vi "Cycling_No_DAQ_Tasks_RT - cOver100.vi"() -> ()   [LabVIEW 2020]
uses:
  Device-Interface-Layer/stop button3.vi
  Device-Interface-Layer/stop button2.vi
  Device-Interface-Layer/stop button1.vi
panel:
  out "Battery 1 Temp":dbl(graph)
  out "Battery 1 Strain":dbl(graph)
  out "Battery 1 Voltage":dbl(graph)
  out "Battery 1 Current":dbl(graph)
  out "Battery 2 Temp":dbl(graph)
  out "Battery 2 Strain":dbl(graph)
  out "Battery 2 Voltage":dbl(graph)
  out "Battery 2 Current":dbl(graph)
  out "Battery 3 Current":dbl(graph)
  out "Battery 3 Voltage":dbl(graph)
  out "Battery 3 Strain":dbl(graph)
  out "Boolean":bool=TRUE
  out "Battery 3 Temp":dbl(graph)
  out "PS Visa Out 3":refnum<visa-resource-name>
  out "PS error out 3":errorcluster
  in  "PS error in 3":errorcluster caption="PS error in (no error)"
  out "PS Visa Out 2":refnum<visa-resource-name>
  out "PS error out 2":errorcluster
  in  "PS error in 2":errorcluster caption="PS error in (no error)"
  out "PS error out":errorcluster
  out "PS Visa Out":refnum<visa-resource-name>
  in  "PS error in":errorcluster caption="PS error in (no error)"
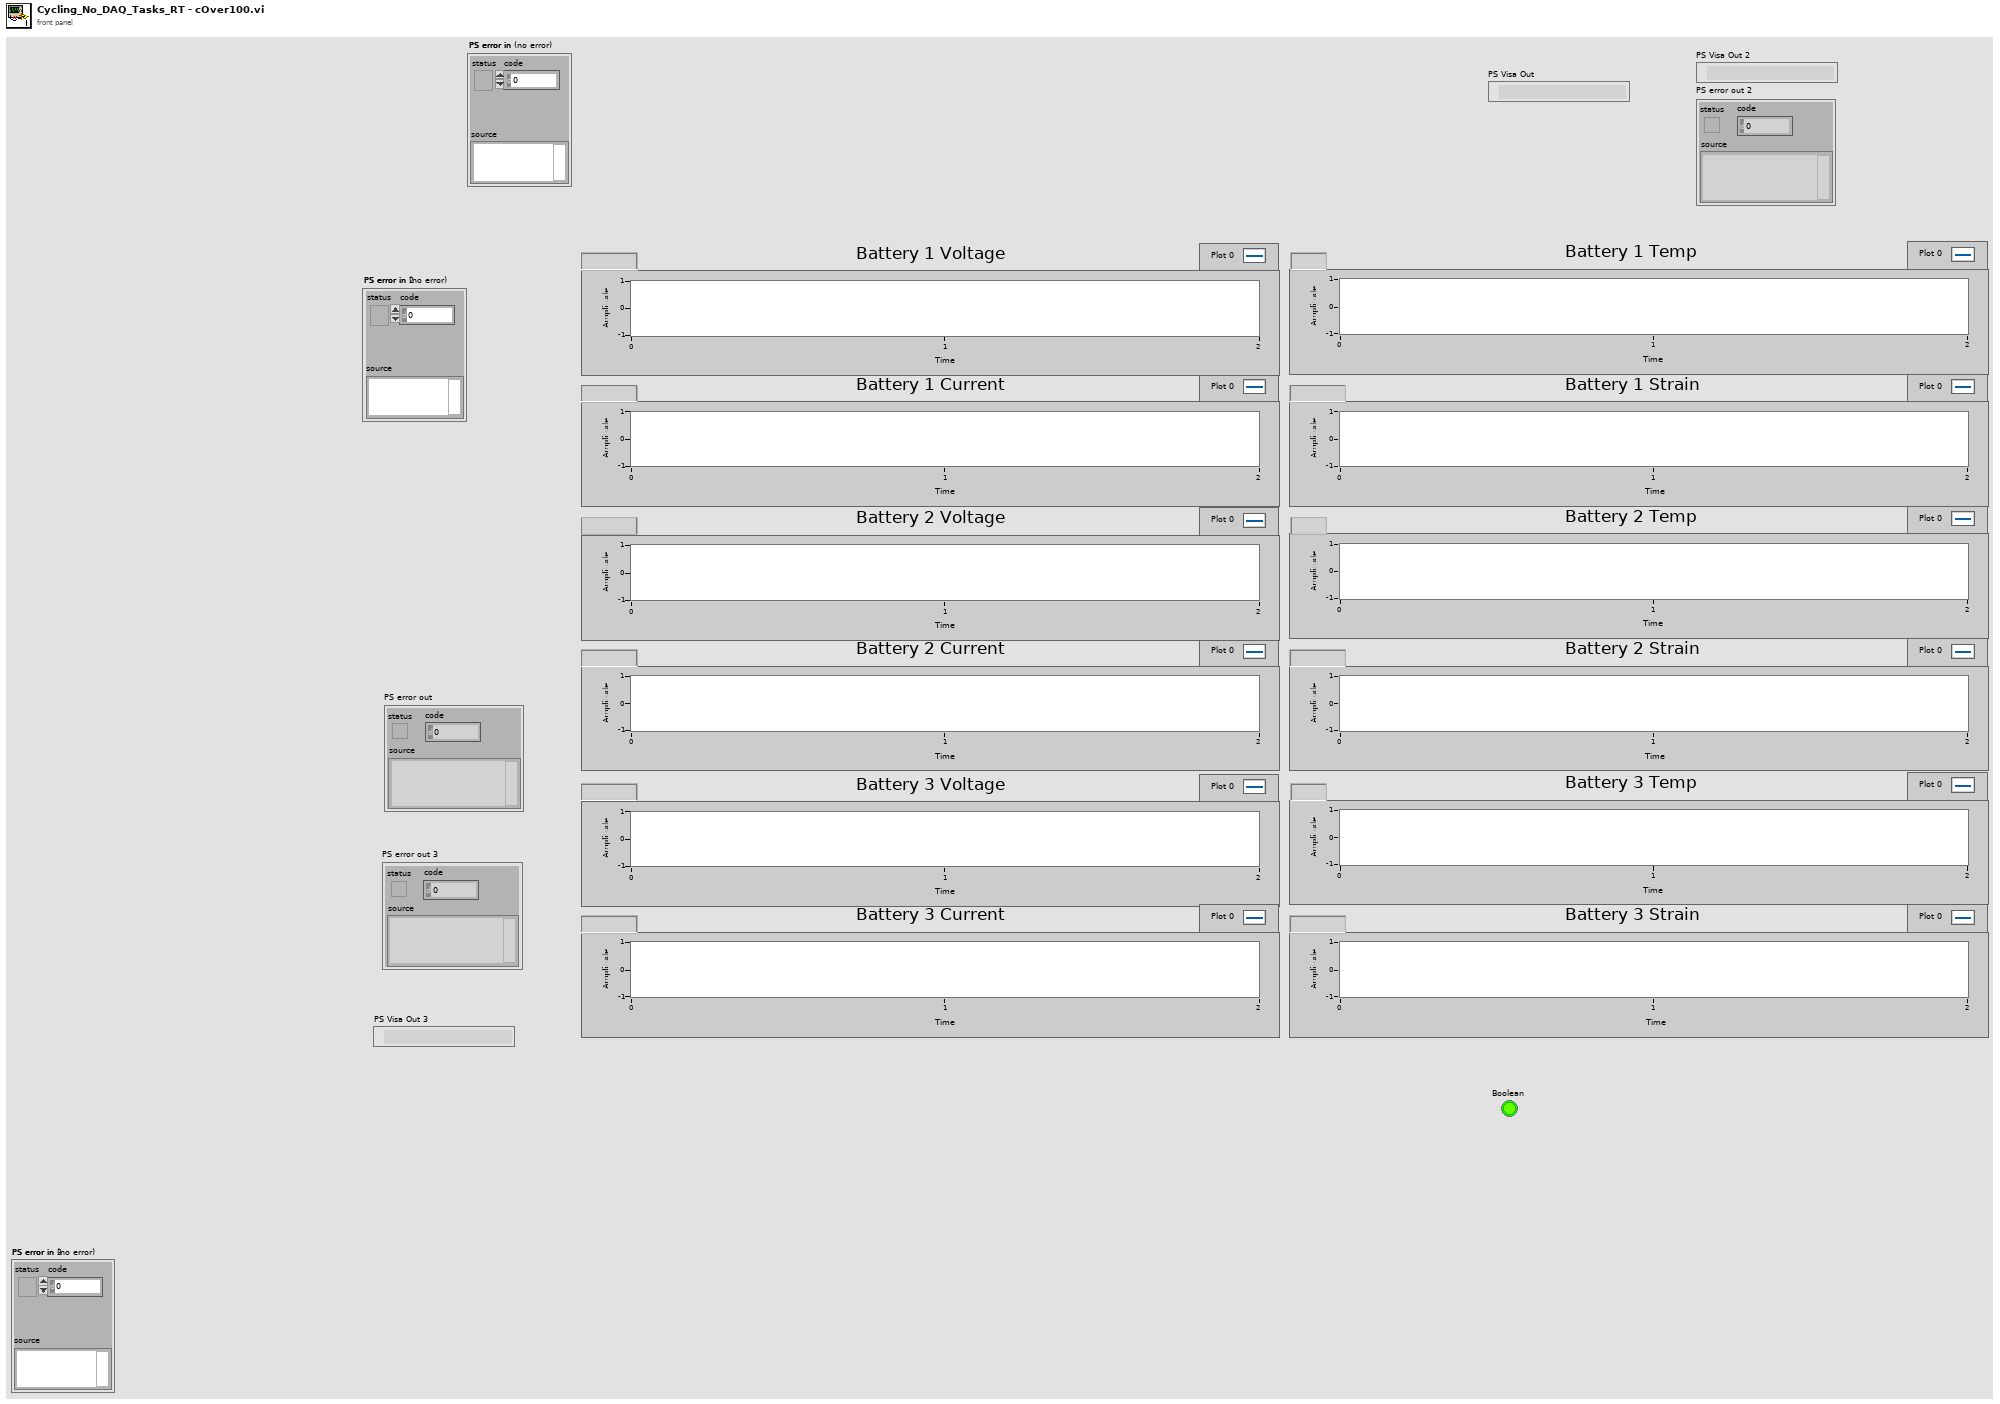
[diagram p1: front panel]
types:
  T1 = enum16{"\"30Q\"", "\"40T\"", "\"2P30Q\"", "\"3P30Q\"", "\"Nissan Leaf\""}
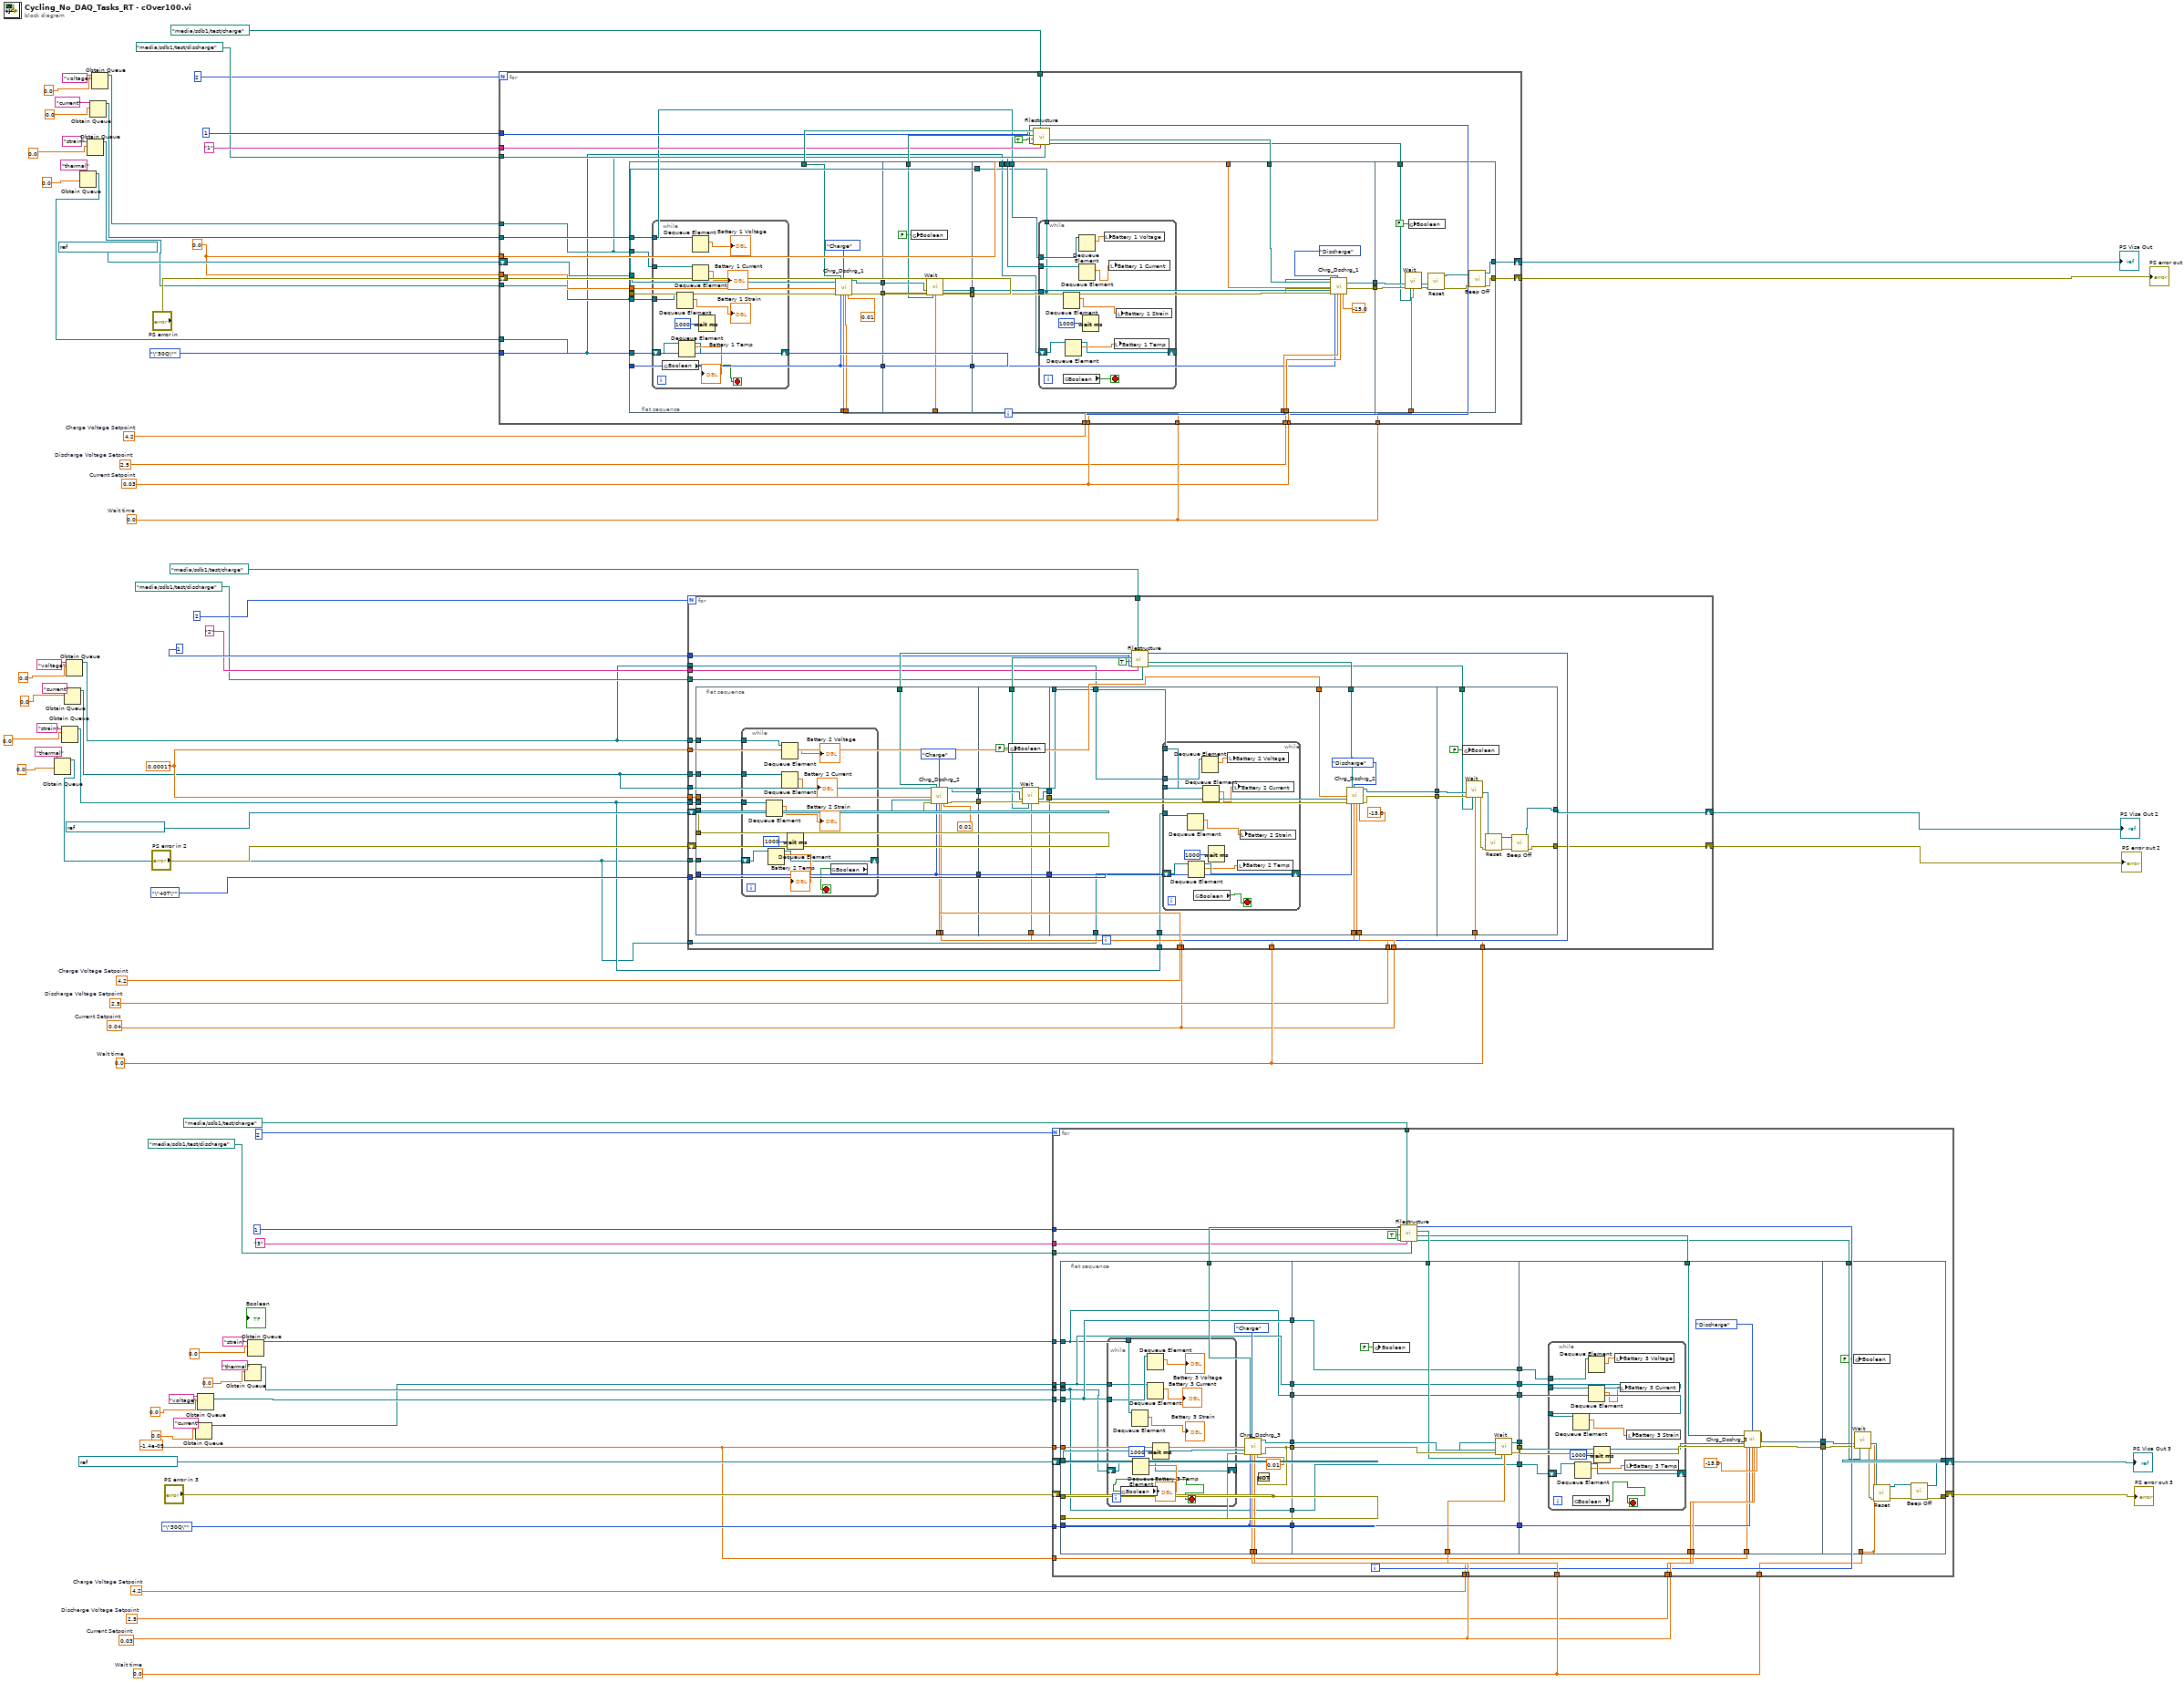
[diagram p0: block diagram]
diagram:
  w3 = -1.4e-05 ("Strain Offset")
  w38 = 0.00017 ("Strain Offset")
  w39 = 2.5  # Discharge Voltage Setpoint
  w42 = 0.0  # Wait time
  w40 = 0.03  # Current Setpoint
  w41 = 4.2  # Charge Voltage Setpoint
  w45 = 2.5  # Discharge Voltage Setpoint
  w46 = 0.0  # Wait time
  w44 = 0.04  # Current Setpoint
  w43 = 4.2  # Charge Voltage Setpoint
  w47 = 2.5  # Discharge Voltage Setpoint
  w50 = 0.0 ("Strain Offset")
  w51 = 0.0  # Wait time
  w49 = 0.03  # Current Setpoint
  w48 = 4.2  # Charge Voltage Setpoint
  n1 = Obtain Queue(name (unnamed)="thermal", element data type=0.0) -> (queue out=w4:refnum<queue>)  [unwired: 3 in, 2 out]
  n2 = Obtain Queue(name (unnamed)="strain", element data type=0.0) -> (queue out=w5:refnum<queue>)  [unwired: 3 in, 2 out]
  n3 = Obtain Queue(name (unnamed)="current", element data type=0.0) -> (queue out=w6:refnum<queue>)  [unwired: 3 in, 2 out]
  n4 = Obtain Queue(name (unnamed)="voltage", element data type=0.0) -> (queue out=w7:refnum<queue>)  [unwired: 3 in, 2 out]
  n5 = Obtain Queue(name (unnamed)="thermal", element data type=0.0) -> (queue out=w8:refnum<queue>)  [unwired: 3 in, 2 out]
  n6 = Obtain Queue(name (unnamed)="strain", element data type=0.0) -> (queue out=w9:refnum<queue>)  [unwired: 3 in, 2 out]
  n7 = Obtain Queue(name (unnamed)="current", element data type=0.0) -> (queue out=w10:refnum<queue>)  [unwired: 3 in, 2 out]
  n8 = Obtain Queue(name (unnamed)="voltage", element data type=0.0) -> (queue out=w11:refnum<queue>)  [unwired: 3 in, 2 out]
  n9 = Obtain Queue(name (unnamed)="current", element data type=0.0) -> (queue out=w30:refnum<queue>)  [unwired: 3 in, 2 out]
  n10 = Obtain Queue(name (unnamed)="voltage", element data type=0.0) -> (queue out=w31:refnum<queue>)  [unwired: 3 in, 2 out]
  n11 = Obtain Queue(name (unnamed)="thermal", element data type=0.0) -> (queue out=w36:refnum<queue>)  [unwired: 3 in, 2 out]
  n12 = Obtain Queue(name (unnamed)="strain", element data type=0.0) -> (queue out=w34:refnum<queue>)  [unwired: 3 in, 2 out]
  n13 = for {
    N: 2 ("Number of Cycles") -> [_]
    tunnel: T1."\"30Q\"" ("Battery Type") -> [w106]
    tunnel: w48 -> [w105]
    tunnel: w49 -> [w104]
    tunnel: w51 -> [w92]
    shift-right: [w83] -> w78
    shift-left: refnum<visa-resource-name> "TCPIP0::192.168.0.246::inst0::INSTR" ("PS VISA in") -> [w108]
    shift-right: [w82] -> w79
    shift-left: "PS error in" -> [w107]
    tunnel: 1 ("Starting Cycle") -> [w98]
    tunnel: "1" ("Batteryname") -> [w96]
    tunnel: path "/media/sdb1/test/discharge" ("Discharge filepath") -> [w95]
    tunnel: path "/media/sdb1/test/charge" ("Charge filepath") -> [w94]
    tunnel: w51 -> [w93]
    tunnel: w50 -> [w91]
    tunnel: w50 -> [w90]
    tunnel: w49 -> [w89]
    tunnel: w47 -> [w88]
    tunnel: w11 -> [w87]
    tunnel: w10 -> [w86]
    tunnel: w9 -> [w85]
    tunnel: w8 -> [w84]
    i -> [w99]
    n14 = flat-sequence {
      tunnel: w108 -> [w125]
      tunnel: w107 -> [w126]
      tunnel: w106 -> [w127]
      tunnel: w105 -> [w122]
      tunnel: [w129] -> w116
      tunnel: [w121] -> w115
      tunnel: [w127] -> w114
      tunnel: w103 -> [w130]
      tunnel: w91 -> [w124]
      tunnel: w89 -> [w123]
      tunnel: w87 -> [w120]
      tunnel: w86 -> [w119]
      tunnel: w85 -> [w118]
      tunnel: w84 -> [w117]
      tunnel: w116 -> [w149]
      tunnel: w115 -> [w148]
      tunnel: [w145] -> w113
      tunnel: [w146] -> w112
      tunnel: w114 -> [w150]
      tunnel: [w150] -> w111
      tunnel: w102 -> [w147]
      tunnel: w92 -> [w144]
      tunnel: w113 -> [w160]
      tunnel: w112 -> [w161]
      tunnel: w111 -> [w162]
      tunnel: w88 -> [w163]
      tunnel: w104 -> [w164]
      tunnel: w101 -> [w159]
      tunnel: [w157] -> w110
      tunnel: [w156] -> w109
      tunnel: w90 -> [w155]
      tunnel: w87 -> [w154]
      tunnel: w86 -> [w153]
      tunnel: w85 -> [w152]
      tunnel: w84 -> [w151]
      tunnel: w100 -> [w182]
      tunnel: w110 -> [w187]
      tunnel: w109 -> [w186]
      tunnel: w93 -> [w183]
      tunnel: [w178] -> w83
      tunnel: [w177] -> w82
      frame #0 {
        n15 = while {
          shift-right: [w140] -> _
          shift-left: w117 -> [w139]
          tunnel: w119 -> [w137]
          tunnel: w120 -> [w134]
          tunnel: w118 -> [w133]
          stop <- w132 stop-if-true
          n16 = global read "stop button1.vi" "Boolean"() -> (w132:bool)
          n17 = Dequeue Element(queue=w133) -> (element=→"Battery 1 Strain":dbl)  [unwired: 2 in, 3 out]
          n18 = Dequeue Element(queue=w139) -> (queue out=w140:refnum<queue>, element=→"Battery 1 Temp":dbl)  [unwired: 2 in, 2 out]
          n19 = Dequeue Element(queue=w134) -> (element=→"Battery 1 Voltage":dbl)  [unwired: 2 in, 3 out]
          n20 = Dequeue Element(queue=w137) -> (element=→"Battery 1 Current":dbl)  [unwired: 2 in, 3 out]
          n21 = Wait (ms)(milliseconds to wait=1000) -> ()  [unwired: 1 out]
        }
        n22 = call "Chrg_Dschrg_1.vi"("Strain Offset"=w124, "PS VISA in"=w125, "PS error in"=w126, "CyclePath"=w130, "Battery Type"=w127, "Charge/discharge"=enum8{"Charge", "Discharge"}."Charge", "Charge/Discharge Voltage Setpoint"=w122, "Current Setpoint"=w123, "Current Cutoff"=0.01) -> ("PS VISA out"=w129:refnum<visa-resource-name>, "PS error out"=w121:errorcluster)  [unwired: 9 in]
      }
      frame #1 {
        n23 = global write "stop button1.vi" "Boolean"(FALSE ("Boolean")) -> ()
        n24 = call "Wait.vi"("PS VISA in"=w149, "PS error in"=w148, "Wait Filepath"=w147, "Wait time"=w144) -> ("PS Visa Out"=w145:refnum<visa-resource-name>, "PS error out"=w146:errorcluster)  [unwired: 10 in]
      }
      frame #2 {
        n25 = while {
          shift-right: [w175] -> _
          shift-left: w151 -> [w174]
          tunnel: [w167] -> _
          tunnel: w153 -> [w173]
          tunnel: w154 -> [w168]
          tunnel: w152 -> [w167]
          stop <- w166 stop-if-true
          n26 = Dequeue Element(queue=w167) -> (element=w170:dbl)  [unwired: 2 in, 3 out]
          n27 = global read "stop button1.vi" "Boolean"() -> (w166:bool)
          n28 = Dequeue Element(queue=w174) -> (queue out=w175:refnum<queue>, element=w169:dbl)  [unwired: 2 in, 2 out]
          n29 = Dequeue Element(queue=w168) -> (element=w172:dbl)  [unwired: 2 in, 3 out]
          n30 = Dequeue Element(queue=w173) -> (element=w171:dbl)  [unwired: 2 in, 3 out]
          n31 = Wait (ms)(milliseconds to wait=1000) -> ()  [unwired: 1 out]
          n32 = local write "Battery 1 Voltage"(w172) -> ()
          n33 = local write "Battery 1 Current"(w171) -> ()
          n34 = local write "Battery 1 Temp"(w169) -> ()
          n35 = local write "Battery 1 Strain"(w170) -> ()
        }
        n36 = call "Chrg_Dschrg_1.vi"("Strain Offset"=w155, "PS VISA in"=w160, "PS error in"=w161, "CyclePath"=w159, "Battery Type"=w162, "Charge/discharge"=enum8{"Charge", "Discharge"}."Discharge", "Charge/Discharge Voltage Setpoint"=w163, "Current Setpoint"=w164, "Current Cutoff"=-15.0) -> ("PS VISA out"=w157:refnum<visa-resource-name>, "PS error out"=w156:errorcluster)  [unwired: 9 in]
      }
      frame #3 {
        n37 = call "Wait.vi"("PS VISA in"=w187, "PS error in"=w186, "Wait Filepath"=w182, "Wait time"=w183) -> ("PS Visa Out"=w185:refnum<visa-resource-name>, "PS error out"=w184:errorcluster)  [unwired: 10 in]
        n38 = global write "stop button1.vi" "Boolean"(FALSE ("Boolean")) -> ()
        n39 = call "Reset.vi"("error in"=w184, "VISA resource name"=w185) -> ("error out"=w179:errorcluster, "VISA resource name out"=w180:refnum<visa-resource-name>)  [unwired: 8 in]
        n40 = call "Beep Off.vi"("error in"=w179, "VISA resource name"=w180) -> ("error out"=w177:errorcluster, "VISA resource name out"=w178:refnum<visa-resource-name>)  [unwired: 8 in]
      }
    }
    n41 = call "Filestructure.vi"("Discharge filepath"=w95, "Batteryname"=w96, "Charge filepath"=w94, "For loop i"=w99, "In for loop"=TRUE, "Starting Cycle"=w98) -> ("DischargeWaitPath"=w100:path, "DischargeCyclePath"=w101:path, "ChargeWaitPath"=w102:path, "ChargeCyclePath"=w103:path)  [unwired: 1 in, 1 out]
  }
  "PS error out" <- w79
  "PS Visa Out" <- w78
  n42 = for {
    N: 2 ("Number of Cycles") -> [_]
    tunnel: T1."\"40T\"" ("Battery Type") -> [w216]
    tunnel: w44 -> [w215]
    tunnel: w44 -> [w214]
    shift-right: [w209] -> w68
    shift-left: refnum<visa-resource-name> "TCPIP0::192.168.0.247::inst0::INSTR" ("PS VISA in") -> [w218]
    shift-right: [w202] -> w69
    shift-left: "PS error in 2" -> [w217]
    tunnel: 1 ("Starting Cycle") -> [w207]
    tunnel: "2" ("Batteryname 2") -> [w205]
    tunnel: path "/media/sdb1/test/discharge" ("Discharge filepath") -> [w204]
    tunnel: path "/media/sdb1/test/charge" ("Charge filepath") -> [w203]
    tunnel: w46 -> [w201]
    tunnel: w46 -> [w200]
    tunnel: w45 -> [w199]
    tunnel: w43 -> [w198]
    tunnel: w38 -> [w197]
    tunnel: w38 -> [w196]
    tunnel: w7 -> [w195]
    tunnel: w6 -> [w194]
    tunnel: w5 -> [w193]
    tunnel: w4 -> [w192]
    tunnel: w7 -> [w191]
    tunnel: w6 -> [w190]
    tunnel: w5 -> [w189]
    tunnel: w4 -> [w188]
    i -> [w208]
    n43 = flat-sequence {
      tunnel: w218 -> [w235]
      tunnel: w217 -> [w236]
      tunnel: w216 -> [w237]
      tunnel: w215 -> [w238]
      tunnel: [w234] -> w226
      tunnel: [w231] -> w225
      tunnel: [w237] -> w224
      tunnel: w213 -> [w240]
      tunnel: w198 -> [w233]
      tunnel: w197 -> [w232]
      tunnel: w195 -> [w230]
      tunnel: w194 -> [w229]
      tunnel: w193 -> [w228]
      tunnel: w192 -> [w227]
      tunnel: w226 -> [w259]
      tunnel: w225 -> [w258]
      tunnel: [w254] -> w223
      tunnel: [w255] -> w222
      tunnel: w224 -> [w260]
      tunnel: [w260] -> w221
      tunnel: w212 -> [w257]
      tunnel: w200 -> [w256]
      tunnel: w223 -> [w270]
      tunnel: w222 -> [w271]
      tunnel: w221 -> [w272]
      tunnel: w199 -> [w273]
      tunnel: w214 -> [w274]
      tunnel: w211 -> [w269]
      tunnel: [w267] -> w220
      tunnel: [w266] -> w219
      tunnel: w196 -> [w265]
      tunnel: w191 -> [w264]
      tunnel: w190 -> [w263]
      tunnel: w189 -> [w262]
      tunnel: w188 -> [w261]
      tunnel: w210 -> [w292]
      tunnel: w220 -> [w297]
      tunnel: w219 -> [w296]
      tunnel: w201 -> [w293]
      tunnel: [w290] -> w209
      tunnel: [w287] -> w202
      frame #0 {
        n44 = while {
          shift-right: [w250] -> _
          shift-left: w227 -> [w249]
          tunnel: w229 -> [w247]
          tunnel: w230 -> [w244]
          tunnel: w228 -> [w243]
          stop <- w242 stop-if-true
          n45 = Dequeue Element(queue=w243) -> (element=→"Battery 2 Strain":dbl)  [unwired: 2 in, 3 out]
          n46 = Dequeue Element(queue=w249) -> (queue out=w250:refnum<queue>, element=→"Battery 2 Temp":dbl)  [unwired: 2 in, 2 out]
          n47 = Dequeue Element(queue=w244) -> (element=→"Battery 2 Voltage":dbl)  [unwired: 2 in, 3 out]
          n48 = Dequeue Element(queue=w247) -> (element=→"Battery 2 Current":dbl)  [unwired: 2 in, 3 out]
          n49 = Wait (ms)(milliseconds to wait=1000) -> ()  [unwired: 1 out]
          n50 = global read "stop button2.vi" "Boolean"() -> (w242:bool)
        }
        n51 = call "Chrg_Dschrg_2.vi"("Strain Offset"=w232, "PS VISA in"=w235, "PS error in"=w236, "CyclePath"=w240, "Battery Type"=w237, "Charge/discharge"=enum8{"Charge", "Discharge"}."Charge", "Charge/Discharge Voltage Setpoint"=w233, "Current Setpoint"=w238, "Current Cutoff"=0.01) -> ("PS VISA out"=w234:refnum<visa-resource-name>, "PS error out"=w231:errorcluster)  [unwired: 9 in]
      }
      frame #1 {
        n52 = global write "stop button2.vi" "Boolean"(FALSE ("Boolean")) -> ()
        n53 = call "Wait.vi"("PS VISA in"=w259, "PS error in"=w258, "Wait Filepath"=w257, "Wait time"=w256) -> ("PS Visa Out"=w254:refnum<visa-resource-name>, "PS error out"=w255:errorcluster)  [unwired: 10 in]
      }
      frame #2 {
        n54 = while {
          shift-right: [w285] -> _
          shift-left: w261 -> [w284]
          tunnel: w262 -> [w283]
          tunnel: [w277] -> _
          tunnel: w264 -> [w278]
          tunnel: w263 -> [w277]
          stop <- w276 stop-if-true
          n55 = Dequeue Element(queue=w283) -> (element=w280:dbl)  [unwired: 2 in, 3 out]
          n56 = Dequeue Element(queue=w284) -> (queue out=w285:refnum<queue>, element=w279:dbl)  [unwired: 2 in, 2 out]
          n57 = global read "stop button2.vi" "Boolean"() -> (w276:bool)
          n58 = Dequeue Element(queue=w278) -> (element=w282:dbl)  [unwired: 2 in, 3 out]
          n59 = Dequeue Element(queue=w277) -> (element=w281:dbl)  [unwired: 2 in, 3 out]
          n60 = Wait (ms)(milliseconds to wait=1000) -> ()  [unwired: 1 out]
          n61 = local write "Battery 2 Voltage"(w282) -> ()
          n62 = local write "Battery 2 Current"(w281) -> ()
          n63 = local write "Battery 2 Temp"(w279) -> ()
          n64 = local write "Battery 2 Strain"(w280) -> ()
        }
        n65 = call "Chrg_Dschrg_2.vi"("Strain Offset"=w265, "PS VISA in"=w270, "PS error in"=w271, "CyclePath"=w269, "Battery Type"=w272, "Charge/discharge"=enum8{"Charge", "Discharge"}."Discharge", "Charge/Discharge Voltage Setpoint"=w273, "Current Setpoint"=w274, "Current Cutoff"=-15.0) -> ("PS VISA out"=w267:refnum<visa-resource-name>, "PS error out"=w266:errorcluster)  [unwired: 9 in]
      }
      frame #3 {
        n66 = global write "stop button2.vi" "Boolean"(FALSE ("Boolean")) -> ()
        n67 = call "Wait.vi"("PS VISA in"=w297, "PS error in"=w296, "Wait Filepath"=w292, "Wait time"=w293) -> ("PS Visa Out"=w295:refnum<visa-resource-name>, "PS error out"=w294:errorcluster)  [unwired: 10 in]
        n68 = call "Reset.vi"("error in"=w294, "VISA resource name"=w295) -> ("error out"=w288:errorcluster, "VISA resource name out"=w289:refnum<visa-resource-name>)  [unwired: 8 in]
        n69 = call "Beep Off.vi"("error in"=w288, "VISA resource name"=w289) -> ("error out"=w287:errorcluster, "VISA resource name out"=w290:refnum<visa-resource-name>)  [unwired: 8 in]
      }
    }
    n70 = call "Filestructure.vi"("Discharge filepath"=w204, "Batteryname"=w205, "Charge filepath"=w203, "For loop i"=w208, "In for loop"=TRUE, "Starting Cycle"=w207) -> ("DischargeWaitPath"=w210:path, "DischargeCyclePath"=w211:path, "ChargeWaitPath"=w212:path, "ChargeCyclePath"=w213:path)  [unwired: 1 in, 1 out]
  }
  "PS error out 2" <- w69
  "PS Visa Out 2" <- w68
  n71 = for {
    N: 2 ("Number of Cycles") -> [_]
    tunnel: T1."\"30Q\"" ("Battery Type") -> [w331]
    tunnel: w40 -> [w330]
    tunnel: w40 -> [w329]
    tunnel: w42 -> [w324]
    shift-right: [w323] -> w58
    shift-left: refnum<visa-resource-name> "TCPIP0::192.168.0.248::inst0::INSTR" ("PS VISA in") -> [w332]
    shift-right: [w316] -> w59
    shift-left: "PS error in 3" -> [w311]
    tunnel: 1 ("Starting Cycle") -> [w321]
    tunnel: "3" ("Batteryname 3") -> [w319]
    tunnel: path "/media/sdb1/test/discharge" ("Discharge filepath") -> [w318]
    tunnel: path "/media/sdb1/test/charge" ("Charge filepath") -> [w317]
    tunnel: w42 -> [w315]
    tunnel: w41 -> [w314]
    tunnel: w39 -> [w313]
    tunnel: w3 -> [w312]
    tunnel: w36 -> [w310]
    tunnel: w34 -> [w309]
    tunnel: w31 -> [w308]
    tunnel: w30 -> [w307]
    tunnel: w3 -> [w298]
    i -> [w322]
    n72 = flat-sequence {
      tunnel: w332 -> [w348]
      tunnel: w311 -> [w349]
      tunnel: w331 -> [w350]
      tunnel: w330 -> [w351]
      tunnel: [w353] -> w340
      tunnel: [w345] -> w339
      tunnel: [w350] -> w338
      tunnel: w328 -> [w354]
      tunnel: w314 -> [w347]
      tunnel: w312 -> [w346]
      tunnel: w311 -> [_]
      tunnel: w310 -> [w341]
      tunnel: w309 -> [w342]
      tunnel: w308 -> [w344]
      tunnel: w307 -> [w343]
      tunnel: [w344] -> w306
      tunnel: [w343] -> w305
      tunnel: [w342] -> w304
      tunnel: [w341] -> w303
      tunnel: w340 -> [w377]
      tunnel: w339 -> [w376]
      tunnel: [w372] -> w337
      tunnel: [w373] -> w336
      tunnel: w338 -> [w378]
      tunnel: [w378] -> w335
      tunnel: w327 -> [w375]
      tunnel: w324 -> [w374]
      tunnel: w306 -> [w371]
      tunnel: w305 -> [w370]
      tunnel: w304 -> [w369]
      tunnel: w303 -> [w368]
      tunnel: [w371] -> w302
      tunnel: [w370] -> w301
      tunnel: [w369] -> w300
      tunnel: [w368] -> w299
      tunnel: w337 -> [w388]
      tunnel: w336 -> [w389]
      tunnel: w335 -> [w390]
      tunnel: w313 -> [w391]
      tunnel: w329 -> [w392]
      tunnel: w326 -> [w387]
      tunnel: [w385] -> w334
      tunnel: [w384] -> w333
      tunnel: w302 -> [w383]
      tunnel: w301 -> [w382]
      tunnel: w300 -> [w381]
      tunnel: w299 -> [w380]
      tunnel: w298 -> [w379]
      tunnel: w325 -> [w411]
      tunnel: w334 -> [w415]
      tunnel: w333 -> [w414]
      tunnel: [w410] -> _
      tunnel: [w408] -> w323
      tunnel: [w405] -> w316
      tunnel: w315 -> [w410]
      frame #0 {
        n73 = while {
          shift-right: [w364] -> _
          shift-left: w341 -> [w363]
          tunnel: w342 -> [w362]
          tunnel: w344 -> [w360]
          tunnel: w343 -> [w359]
          stop <- w356 stop-if-true
          n74 = global read "stop button3.vi" "Boolean"() -> (w356:bool)
          n75 = Dequeue Element(queue=w362) -> (element=→"Battery 3 Strain":dbl)  [unwired: 2 in, 3 out]
          n76 = Dequeue Element(queue=w363) -> (queue out=w364:refnum<queue>, element=→"Battery 3 Temp":dbl)  [unwired: 2 in, 2 out]
          n77 = Dequeue Element(queue=w360) -> (element=→"Battery 3 Voltage":dbl)  [unwired: 2 in, 3 out]
          n78 = Dequeue Element(queue=w359) -> (element=→"Battery 3 Current":dbl)  [unwired: 2 in, 3 out]
          n79 = Wait (ms)(milliseconds to wait=1000) -> ()  [unwired: 1 out]
        }
        n80 = call "Chrg_Dschrg_3.vi"("Strain Offset"=w346, "PS VISA in"=w348, "PS error in"=w349, "CyclePath"=w354, "Battery Type"=w350, "Charge/discharge"=enum8{"Charge", "Discharge"}."Charge", "Charge/Discharge Voltage Setpoint"=w347, "Current Setpoint"=w351, "Current Cutoff"=0.01) -> ("PS VISA out"=w353:refnum<visa-resource-name>, "PS error out"=w345:errorcluster)  [unwired: 9 in]
        n81 = Not(x=w345) -> ()  [unwired: 1 out]
      }
      frame #1 {
        n82 = global write "stop button3.vi" "Boolean"(FALSE ("Boolean")) -> ()
        n83 = call "Wait.vi"("PS VISA in"=w377, "PS error in"=w376, "Wait Filepath"=w375, "Wait time"=w374) -> ("PS Visa Out"=w372:refnum<visa-resource-name>, "PS error out"=w373:errorcluster)  [unwired: 10 in]
      }
      frame #2 {
        n84 = while {
          shift-right: [w403] -> _
          shift-left: w380 -> [w402]
          tunnel: w381 -> [w401]
          tunnel: w382 -> [w400]
          tunnel: w383 -> [w395]
          stop <- w394 stop-if-true
          n85 = Dequeue Element(queue=w401) -> (element=w397:dbl)  [unwired: 2 in, 3 out]
          n86 = global read "stop button3.vi" "Boolean"() -> (w394:bool)
          n87 = Dequeue Element(queue=w402) -> (queue out=w403:refnum<queue>, element=w396:dbl)  [unwired: 2 in, 2 out]
          n88 = Dequeue Element(queue=w395) -> (element=w399:dbl)  [unwired: 2 in, 3 out]
          n89 = Dequeue Element(queue=w400) -> (element=w398:dbl)  [unwired: 2 in, 3 out]
          n90 = Wait (ms)(milliseconds to wait=1000) -> ()  [unwired: 1 out]
          n91 = local write "Battery 3 Voltage"(w399) -> ()
          n92 = local write "Battery 3 Current"(w398) -> ()
          n93 = local write "Battery 3 Temp"(w396) -> ()
          n94 = local write "Battery 3 Strain"(w397) -> ()
        }
        n95 = call "Chrg_Dschrg_3.vi"("Strain Offset"=w379, "PS VISA in"=w388, "PS error in"=w389, "CyclePath"=w387, "Battery Type"=w390, "Charge/discharge"=enum8{"Charge", "Discharge"}."Discharge", "Charge/Discharge Voltage Setpoint"=w391, "Current Setpoint"=w392, "Current Cutoff"=-15.0) -> ("PS VISA out"=w385:refnum<visa-resource-name>, "PS error out"=w384:errorcluster)  [unwired: 9 in]
      }
      frame #3 {
        n96 = global write "stop button3.vi" "Boolean"(FALSE ("Boolean")) -> ()
        n97 = call "Wait.vi"("PS VISA in"=w415, "PS error in"=w414, "Wait Filepath"=w411, "Wait time"=w410) -> ("PS Visa Out"=w413:refnum<visa-resource-name>, "PS error out"=w412:errorcluster)  [unwired: 10 in]
        n98 = call "Reset.vi"("error in"=w412, "VISA resource name"=w413) -> ("error out"=w406:errorcluster, "VISA resource name out"=w407:refnum<visa-resource-name>)  [unwired: 8 in]
        n99 = call "Beep Off.vi"("error in"=w406, "VISA resource name"=w407) -> ("error out"=w405:errorcluster, "VISA resource name out"=w408:refnum<visa-resource-name>)  [unwired: 8 in]
      }
    }
    n100 = call "Filestructure.vi"("Discharge filepath"=w318, "Batteryname"=w319, "Charge filepath"=w317, "For loop i"=w322, "In for loop"=TRUE, "Starting Cycle"=w321) -> ("DischargeWaitPath"=w325:path, "DischargeCyclePath"=w326:path, "ChargeWaitPath"=w327:path, "ChargeCyclePath"=w328:path)  [unwired: 1 in, 1 out]
  }
  "PS error out 3" <- w59
  "PS Visa Out 3" <- w58
